vi "Dispose.vi"(8 "error in (no error)":errorcluster, 11 "Pub Sub Retaining Message Channel in":refnum<class "Pub Sub Retaining Message Channel.lvclass">) -> (0 "error out":errorcluster, 3 "Pub Sub Retaining Message Channel in 2":refnum<class "Pub Sub Retaining Message Channel.lvclass">)   [LabVIEW 2020, in "Actor Pub Sub Channels.lvlib" / "Pub Sub Retaining Message Channel.lvclass"]
uses:
  Pub Sub Retaining Message Channel.lvclass
  Pub Sub Retaining Message Channel.lvclass/Pub Sub Retaining Message Channel.ctl
  Pub Sub Message Channel/Pub Sub Message Channel.lvclass
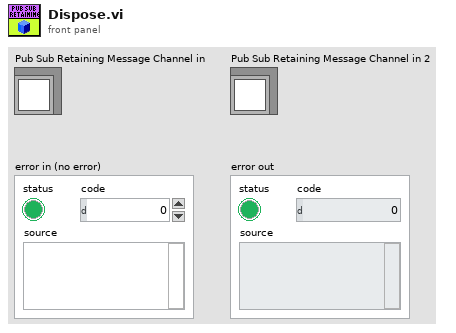
[diagram p1: front panel]
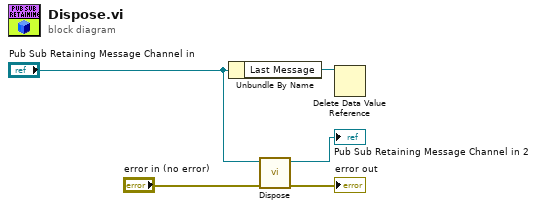
[diagram p0: block diagram]
diagram:
  n1 = Unbundle By Name("Pub Sub Retaining Message Channel in") -> ("Last Message"=w1:refnum<data-value>)
  n2 = call-parent "Dispose.vi"("error in (no error)"="error in (no error)", "Pub Sub Message Channel in"="Pub Sub Retaining Message Channel in") -> ("error out"=→"error out":errorcluster, "Pub Sub Message Channel in 2"=→"Pub Sub Retaining Message Channel in 2":refnum<class "Pub Sub Retaining Message Channel.lvclass">)  [unwired: 8 in]
  n3 = Delete Data Value Reference(data value reference=w1) -> ()  [unwired: 1 in, 2 out]
